vi "dfd_FXP Quantization (scaler).vi"(4 "quantization settings":T1={"source"=6, "wl"=1, "iwl"=1, "overflow mode"=enum."Saturation", "rounding mode"=enum."Nearest", "signed?"=TRUE} {"source" items=["Coef a/k"=0, "Coef b/v"=7, "Input"=1, "Output"=2, "Multiplicand"=3, "Product"=4, "Sum"=5, "Delay"=6, "Gain"=8]}, 8 "value in":dbl format="%.2f") -> (3 "value out":dbl format="%.2f")   [LabVIEW 2017, in "NI_DigFilter_FXP.lvlib"]
uses:
  <vilib>/addons/Digital Filter Design/NI_DigFilter_FXP.lvlib
  <vilib>/addons/Digital Filter Design/_Objects.llb/dfd_Internal Quantization Settings.ctl
  <vilib>/addons/Digital Filter Design/_Objects.llb/dfd_Internal Quantization Srcs.ctl
  <vilib>/addons/Digital Filter Design/NI_DigFilterLicensed.lvlib
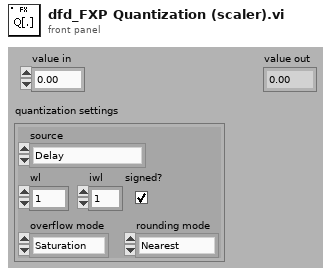
[diagram p1: front panel]
types:
  T1 = typedef "NI_DigFilterLicensed.lvlib/dfd_Internal Quantization Settings.ctl" = cluster{"source":T2, "wl":i16, "iwl":i16, "overflow mode":enum16{"Saturation", "Wrap"}, "rounding mode":enum16{"Nearest", "Truncation"}, "signed?":bool}
  T2 = typedef "NI_DigFilterLicensed.lvlib/dfd_Internal Quantization Srcs.ctl" = u16
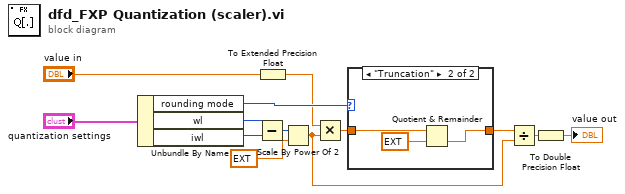
[diagram p0: block diagram]
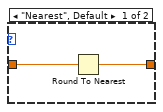
[diagram p2: hidden frame]
diagram:
  n1 = Unbundle By Name("quantization settings") -> ("rounding mode"=w3:enum16{"Nearest", "Truncation"}, "wl"=w13:i16, "iwl"=w12:i16)
  n2 = Subtract(x=w13, y=w12) -> (x-y=w11:i16)
  n3 = To Extended Precision Float(1:"value in") -> (0:w1:ext)
  n4 = Scale By Power Of 2(n=w11, x=ext 1.0) -> (x*2^n=w7:ext)
  n5 = Multiply(x=w1, y=w7) -> (x*y=w9:ext)
  n6 = case shown="\"Truncation\"" w3 {
    tunnel: w9 -> [w15 w18]
    tunnel: [w14 w16] -> w8
    frame "Nearest", Default {
      n7 = Round To Nearest(number=w15) -> (nearest integer value=w14:ext)
    }
    frame "Truncation" {
      n8 = Quotient & Remainder(x=w18, y=ext 1.0) -> (floor(x/y)=w16:ext)  [unwired: 1 out]
    }
  }
  n9 = Divide(x=w8, y=w7) -> (x/y=w5:ext)
  n10 = To Double Precision Float(number=w5) -> (double precision float=→"value out":dbl)
